vi "Sort1DWithSortMap.vi"(1 "Original":dbl[](array[numeric]), 2 "Sort Map":T1(array[cluster])) -> (0 "Sorted":dbl[](array[numeric]))   [LabVIEW 2010]
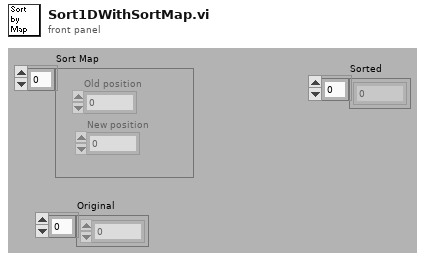
[diagram p1: front panel]
types:
  T1 = cluster{"Old position":dbl, "New position":dbl}[]
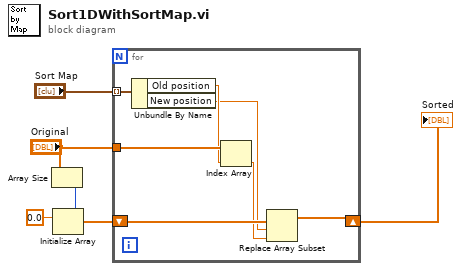
[diagram p0: block diagram]
diagram:
  n1 = Array Size(array="Original") -> (size(s)=w5:i32)
  n2 = Initialize Array(0.0 ("element"), w5) -> (w3:dbl[])
  n3 = for {
    tunnel: "Sort Map" -> [w13] mode=indexing
    shift-right: [w7] -> w1
    shift-left: w3 -> [w10]
    tunnel: "Original" -> [w12]
    n4 = Unbundle By Name(w13) -> ("Old position"=w11:dbl, "New position"=w8:dbl)
    n5 = Index Array(array=w12, index=w11) -> (element=w9:dbl)
    n6 = Replace Array Subset(array=w10, new element=w9, index=w8) -> (w7:dbl[])
  }
  "Sorted" <- w1
